vi "AVD Threshold.vi"(8 "Cal":string, 9 "Threshol values":dbl[](array[numeric]), 10 "Voltage steps":dbl[](array[numeric]), 11 "AVD curve":dbl[](array[numeric])) -> (1 "pressures":dbl[](array[numeric]) format="%_6g", 3 "Array out":dbl[][](array[numeric]))   [LabVIEW 2022 SP3]
uses:
  <vilib>/gmath/NI_Gmath.lvlib
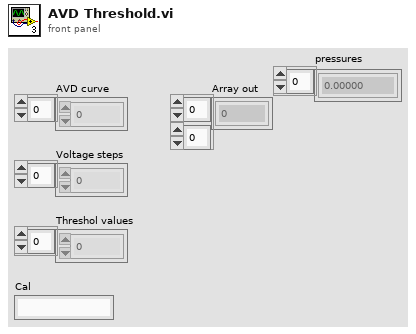
[diagram p1: front panel]
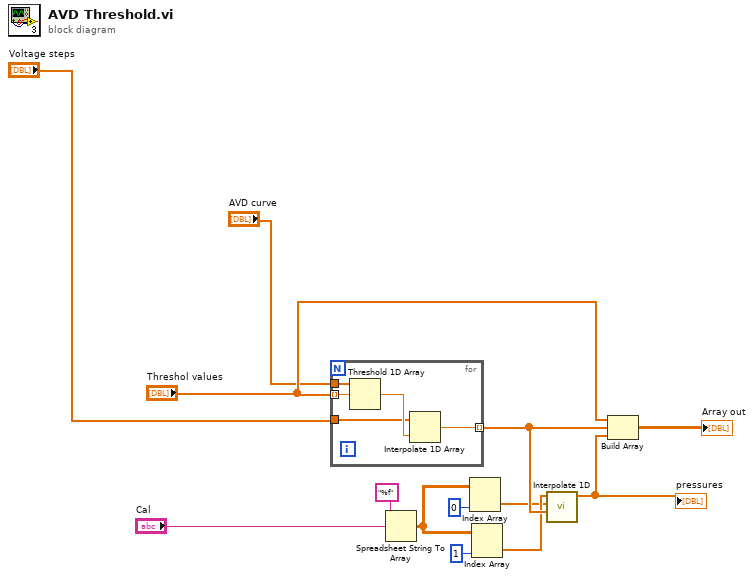
[diagram p0: block diagram]
diagram:
  n1 = for {
    tunnel: "AVD curve" -> [w17]
    tunnel: "Threshol values" -> [w16] mode=indexing
    tunnel: "Voltage steps" -> [w15]
    tunnel: [w14] -> w9 mode=indexing
    n2 = Threshold 1D Array(2:w16, 3:w17) -> (0:w18:dbl)  [unwired: 1 in]
    n3 = Interpolate 1D Array(1:w18, 2:w15) -> (0:w14:dbl)
  }
  n4 = Spreadsheet String To Array(format string="%f", spreadsheet string="Cal") -> (array=w6:dbl[][])  [unwired: 2 in]
  n5 = Index Array(array=w6, index (col)=0 ("disabled index (col)")) -> (element=w7:dbl[])  [unwired: 1 in]
  n6 = Index Array(array=w6, index (col)=1 ("disabled index (col)")) -> (element=w8:dbl[])  [unwired: 1 in]
  n7 = call <vilib>:"Interpolate 1D.vi"("xi"=w9, "X"=w7, "Y"=w8) -> ("yi"=w12:dbl[])  [unwired: 6 in, 2 out]
  "pressures" <- w12
  n8 = Build Array("Threshol values", w9, w12) -> (→"Array out":dbl[][])
